vi "Test Validate File.vi"(4 "error in (no error)":errorcluster, 5 "Test Filename Extension (\"\")":string, 6 "Test Filename w/o Extension (\"\")":string, 7 "Tests Folder (Empty)":path) -> (0 "error out":errorcluster, 1 "Valid?":bool, 2 "Fields":T1[](array[typedef]), 3 "Test Record":T4)   [LabVIEW 2011]
uses:
  Test Record.ctl
  Fields/Field Record.ctl
  Fields/Field DataTypes.ctl
  Fields/Field NextItem.ctl
  Summitek EXT/Miscellaneous/OGAB Version.ctl
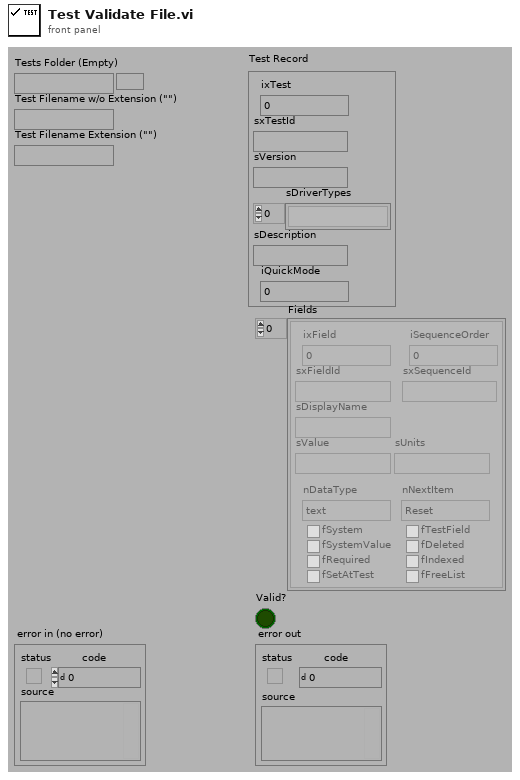
[diagram p1: front panel]
types:
  T1 = typedef "Field Record.ctl" = cluster{"ixField":i32, "iSequenceOrder":i32, "sxFieldId":string, "sxSequenceId":string, "sDisplayName":string, "sValue":string, "sUnits":string, "nDataType":T2, "nNextItem":T3, "fSystem":bool, "fSystemValue":bool, "fRequired":bool, "fSetAtTest":bool, "fTestField":bool, "fDeleted":bool, "fIndexed":bool, "fFreeList":bool}
  T2 = typedef "Field DataTypes.ctl" = enum32{"text", "numeric", "list", "timestamp", "boolean"}
  T3 = typedef "Field NextItem.ctl" = enum32{"Reset", "Retain", "Auto-Increment"}
  T4 = typedef "Test Record.ctl" = cluster{"ixTest":i32, "sxTestId":string, "sVersion":string, "sDriverTypes":string[], "sDescription":string, "iQuickMode":i32}
  T5 = enum32{"invalid app kind", "Development System", "Run Time System", "Student Edition", "Embedded LabVIEW", "Evaluation", "Custom"}
  T6 = typedef "OGAB Version.ctl" = cluster{"Version":string, "Build Number":u32, "Build Date/Time":dbl}
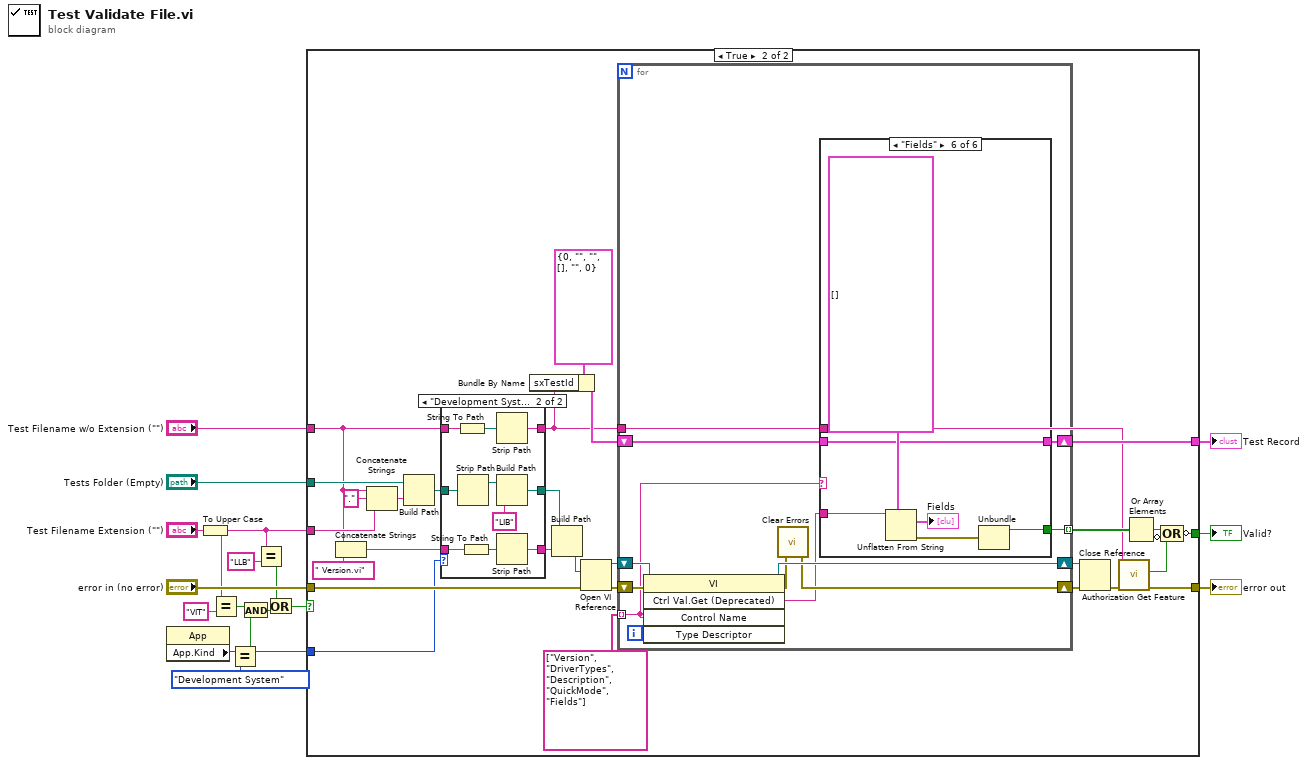
[diagram p0: block diagram]
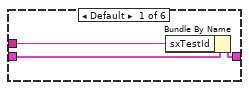
[diagram p4: hidden frame]
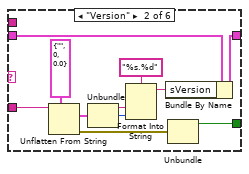
[diagram p5: hidden frame]
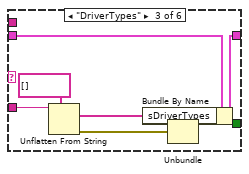
[diagram p6: hidden frame]
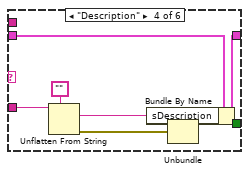
[diagram p7: hidden frame]
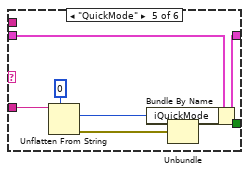
[diagram p8: hidden frame]
diagram:
  n1 = property class="App"() -> ("App.Kind"=w2:T5)  [unwired: 2 in, 2 out]
  n2 = To Upper Case(1:"Test Filename Extension (\"\")") -> (0:w5:string)
  n3 = Equal?(x=w5, y="VIT") -> (x = y?=w8:bool)
  n4 = Equal?(x=w2, y=T5."Development System") -> (x = y?=w3:bool)
  n5 = And(x=w8, y=w3) -> (x .and. y?=w7:bool)
  n6 = Equal?(x=w5, y="LLB") -> (x = y?=w6:bool)
  n7 = Or(x=w6, y=w7) -> (x .or. y?=w4:bool)
  n8 = case shown="True" w4 {
    tunnel: "error in (no error)" -> [w18 w46]
    tunnel: "Tests Folder (Empty)" -> [_ w45]
    tunnel: "Test Filename w/o Extension (\"\")" -> [_ w20]
    tunnel: [_ w42] -> w12
    tunnel: [w18 w29] -> w11
    tunnel: w5 -> [_ w43]
    tunnel: w2 -> [_ w27]
    tunnel: [_ w21] -> w1
    frame False {
    }
    frame True {
      n9 = Concatenate Strings(w20, " Version.vi") -> (w32:string)
      n10 = Concatenate Strings(w20, "." ("string"), w43) -> (w44:string)
      n11 = Build Path(base path=w45, name or relative path=w44) -> (appended path=w34:path)
      n12 = case shown="\"Development System\"" w27 {
        tunnel: w34 -> [w49 w58]
        tunnel: [w49 w56] -> w33
        tunnel: w32 -> [w48 w55]
        tunnel: [w48 w53] -> w31
        tunnel: w20 -> [w47 w52]
        tunnel: [w47 w50] -> w19
        frame Default {
        }
        frame "Development System" {
          n13 = String To Path(string=w52) -> (path=w51:path)
          n14 = Strip Path(path=w58) -> (stripped path=w57:path)  [unwired: 1 out]
          n15 = String To Path(string=w55) -> (path=w54:path)
          n16 = Strip Path(path=w51) -> (name=w50:string)  [unwired: 1 out]
          n17 = Build Path(base path=w57, name or relative path="LIB") -> (appended path=w56:path)
          n18 = Strip Path(path=w54) -> (name=w53:string)  [unwired: 1 out]
        }
      }
      n19 = Bundle By Name(cluster=T4 {"ixTest"=0, "sxTestId"="", "sVersion"="", "sDriverTypes"=[], "sDescription"="", "iQuickMode"=0} ("Test Record"), "sxTestId"=w19) -> (w24:T4)
      n20 = Build Path(base path=w33, name or relative path=w31) -> (appended path=w41:path)
      n21 = Open VI Reference(vi path=w41, error in (no error)=w46) -> (vi reference=w39:refnum<vi>, error out=w38:errorcluster)  [unwired: 4 out]
      n22 = for {
        shift-right: [w69] -> w36
        shift-left: w39 -> [w70]
        shift-right: [w66] -> w35
        shift-left: w38 -> [w68]
        tunnel: string[] ["Version", "DriverTypes", "Description", "QuickMode", "Fields"] -> [w63] mode=indexing
        shift-right: [w64] -> w21
        shift-left: w24 -> [w65]
        tunnel: [w61] -> w23 mode=indexing
        tunnel: w19 -> [w60]
        n23 = invoke class="VI" method="Ctrl Val.Get (Deprecated)"(reference=w70, error in=w68, "Control Name"=w63) -> (reference out=w69:refnum<vi>, error out=w67:errorcluster, "Get Control Value"=w62:string)  [unwired: 2 in, 2 out]
        n24 = call <vilib>:"Clear Errors.vi"("error in (no error)"=w67) -> ("error out"=w66:errorcluster)  [unwired: 6 out]
        n25 = case shown="\"Fields\"" w63 {
          tunnel: w65 -> [w73 w84 w91 w98 w105 w107]
          tunnel: [w72 w83 w90 w97 w104 w107] -> w64
          tunnel: w62 -> [_ w76 w89 w96 w103 w111]
          tunnel: [_ w74 w87 w94 w101 w109] -> w61
          tunnel: w60 -> [w71 _ _ _ _ _]
          frame Default {
            n26 = Bundle By Name(cluster=w73, "sxTestId"=w71) -> (w72:T4)
          }
          frame "Version" {
            n27 = Unflatten From String(type=T6 {"Version"="", "Build Number"=0, "Build Date/Time"=0.0} ("Version"), binary string=w76) -> (value=w80:T6, error out=w75:errorcluster)  [unwired: 1 in, 3 out]
            n28 = Unbundle(w80) -> ("Version"=w81:string, "Build Number"=w82:u32)  [unwired: 1 out]
            n29 = Format Into String(format string="%s.%d", w81, w82) -> (resulting string=w77:string)  [unwired: 2 in, 1 out]
            n30 = Bundle By Name(cluster=w84, "sVersion"=w77) -> (w83:T4)
            n31 = Unbundle(w75) -> ("status"=w74:bool)  [unwired: 2 out]
          }
          frame "DriverTypes" {
            n32 = Unflatten From String(type=string[] [], binary string=w89) -> (value=w85:string[], error out=w88:errorcluster)  [unwired: 1 in, 3 out]
            n33 = Bundle By Name(cluster=w91, "sDriverTypes"=w85) -> (w90:T4)
            n34 = Unbundle(w88) -> ("status"=w87:bool)  [unwired: 2 out]
          }
          frame "Description" {
            n35 = Unflatten From String(type="", binary string=w96) -> (value=w93:string, error out=w95:errorcluster)  [unwired: 1 in, 3 out]
            n36 = Bundle By Name(cluster=w98, "sDescription"=w93) -> (w97:T4)
            n37 = Unbundle(w95) -> ("status"=w94:bool)  [unwired: 2 out]
          }
          frame "QuickMode" {
            n38 = Unflatten From String(type=0, binary string=w103) -> (value=w99:i32, error out=w102:errorcluster)  [unwired: 1 in, 3 out]
            n39 = Bundle By Name(cluster=w105, "iQuickMode"=w99) -> (w104:T4)
            n40 = Unbundle(w102) -> ("status"=w101:bool)  [unwired: 2 out]
          }
          frame "Fields" {
            n41 = Unflatten From String(type=T1[] [], binary string=w111) -> (value=→"Fields":T1[], error out=w110:errorcluster)  [unwired: 1 in, 3 out]
            n42 = Unbundle(w110) -> ("status"=w109:bool)  [unwired: 2 out]
          }
        }
      }
      n43 = Close Reference(reference=w36, error in (no error)=w35) -> (error out=w30:errorcluster)
      n44 = call "Authorization Get Feature.vi"("error in (no error)"=w30, "Feature Name"=w19) -> ("error out"=w29:errorcluster, "Authorized?"=w28:bool)  [unwired: 7 in, 1 out]
      n45 = Or Array Elements(Boolean array=w23) -> (logical OR=w22:bool)
      n46 = Compound Arithmetic op=OR(w22, invert w28) -> (invert w42:bool)
    }
  }
  "error out" <- w11
  "Valid?" <- w12
  "Test Record" <- w1
